vi "_Get FPGA Info.vi"(4 "error in":errorcluster) -> (0 "error out":errorcluster, 3 "Info":string)   [LabVIEW 2012]
uses:
  _RT Global.vi
  <vilib>/Utility/error.llb/Error Cluster From Error Code.vi
  <vilib>/rvi/errors/niLvFpgaAdjustHostInterfaceError.vi
  <vilib>/rvi/interface/nirviReadWriteControl/nirviReadWriteControl.xnode
  FPGA Bitfiles/FPGA9602.lvbitx
  NiFpgaLv.dll
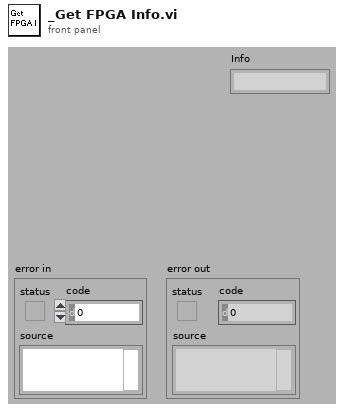
[diagram p1: front panel]
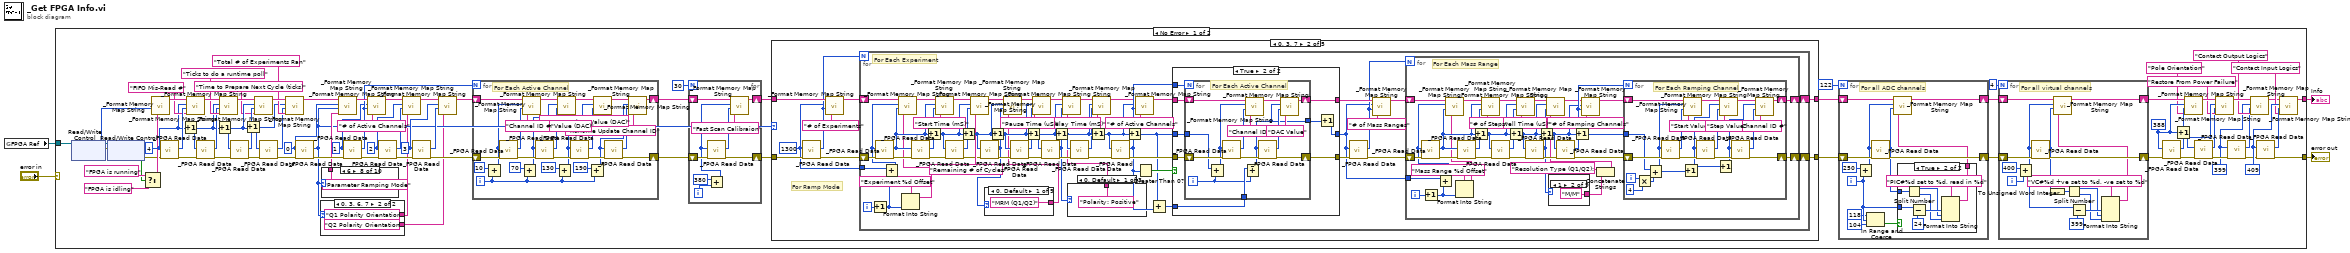
[diagram p0: block diagram]
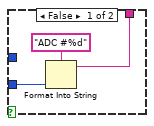
[diagram p2: hidden frame]
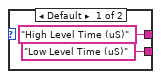
[diagram p3: hidden frame]
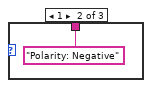
[diagram p5: hidden frame]
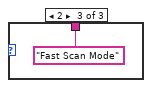
[diagram p6: hidden frame]
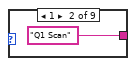
[diagram p7: hidden frame]
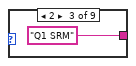
[diagram p8: hidden frame]
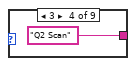
[diagram p9: hidden frame]
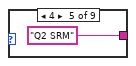
[diagram p10: hidden frame]
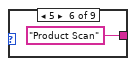
[diagram p11: hidden frame]
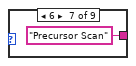
[diagram p12: hidden frame]
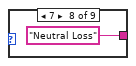
[diagram p13: hidden frame]
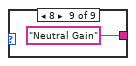
[diagram p14: hidden frame]
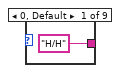
[diagram p15: hidden frame]
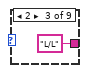
[diagram p16: hidden frame]
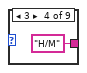
[diagram p17: hidden frame]
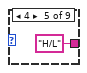
[diagram p18: hidden frame]
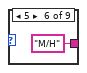
[diagram p19: hidden frame]
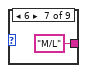
[diagram p20: hidden frame]
diagram:
  n1 = global read "_RT Global.vi" "FPGA Ref"() -> (w1:refnum<k20>)
  n2 = case shown="No Error" "error in" {
    selector: "error in" -> [_ w595]
    tunnel: [w6 w595] -> w3
    tunnel: w1 -> [w82 _]
    tunnel: [w5 _] -> w2
    frame No Error {
      w10 = u16 409 ("Address")
      w13 = u16 399 ("Address")
      w23 = u16 388 ("Address")
      w60 = u16 3 ("Address")
      w55 = u16 2 ("Address")
      w44 = u16 1 ("Address")
      w71 = u16 0 ("Address")
      w74 = u16 4 ("Address")
      n3 = xnode "Read/Write Control"("FPGA VI Reference In"=w82) -> ("FPGA VI Reference Out"=w84:refnum<k20>, "error out"=w83:errorcluster, "Version"=w80:u32)  [unwired: 1 in]
      n4 = xnode "Read/Write Control"("FPGA VI Reference In"=w84, "error in"=w83) -> ("error out"=w79:errorcluster, "Running"=w85:bool)  [unwired: 1 out]
      n5 = Select(t="FPGA is running", s=w85, f="FPGA is idling") -> (s? t:f=w81:string)
      n6 = call "_Format Memory Map String.vi"("User value"=w81, "Data"=w80) -> ("String Out"=w78:string)  [unwired: 2 in, 3 out]
      n7 = call "_FPGA Read Data.vi"("error in"=w79, "Address"=w74) -> ("error out"=w73:errorcluster, "Data"=w77:u32)  [unwired: 3 in, 1 out]
      n8 = Increment(x=w74) -> (x+1=w66:u16)
      n9 = call "_Format Memory Map String.vi"("User value"="FIFO Mis-Read #", "Data"=w77, "Address"=w74, "String In"=w78) -> ("String Out"=w75:string)  [unwired: 3 out]
      n10 = call "_FPGA Read Data.vi"("error in"=w73, "Address"=w66) -> ("error out"=w69:errorcluster, "Data"=w68:u32)  [unwired: 3 in, 1 out]
      n11 = Increment(x=w66) -> (x+1=w64:u16)
      n12 = call "_Format Memory Map String.vi"("User value"="Ticks to do a runtime poll", "Data"=w68, "Address"=w66, "String In"=w75) -> ("String Out"=w70:string)  [unwired: 3 out]
      n13 = call "_FPGA Read Data.vi"("error in"=w69, "Address"=w64) -> ("error out"=w65:errorcluster, "Data"=w67:u32)  [unwired: 3 in, 1 out]
      n14 = Increment(x=w64) -> (x+1=w45:u16)
      n15 = call "_Format Memory Map String.vi"("User value"="Time to Prepare Next Cycle (ticks)", "Data"=w67, "Address"=w64, "String In"=w70) -> ("String Out"=w62:string)  [unwired: 3 out]
      n16 = call "_FPGA Read Data.vi"("error in"=w65, "Address"=w45) -> ("error out"=w42:errorcluster, "Data"=w46:u32)  [unwired: 3 in, 1 out]
      n17 = call "_Format Memory Map String.vi"("User value"="Total # of Experiments Ran", "Data"=w46, "Address"=w45, "String In"=w62) -> ("String Out"=w41:string)  [unwired: 3 out]
      n18 = call "_FPGA Read Data.vi"("error in"=w42, "Address"=w71) -> ("error out"=w50:errorcluster, "Data"=w40:u32)  [unwired: 3 in, 1 out]
      n19 = case shown="0, 3, 6, 7" w40 {
        tunnel: ["High Level Time (uS)" ("User value") "Q1 Polarity Orientation" ("User value")] -> w39
        tunnel: ["Low Level Time (uS)" ("User value") "Q2 Polarity Orientation" ("User value")] -> w38
        frame Default {
        }
        frame 0, 3, 6, 7 {
        }
      }
      n20 = case shown="6" w40 {
        tunnel: ["Unknown Mode" ("User value") "Dual or Ramp Mode" ("User value") "Single Mode" ("User value") "Dual Mode" ("User value") "Ramp Mode" ("User value") "ADC Mode" ("User value") "Oscillator Mode" ("User value") "Parameter Ramping Mode" ("User value") "LC Sync Mode" ("User value") "Set PIC Mode" ("User value")] -> w43
        frame Default {
        }
        frame 0 {
        }
        frame 1 {
        }
        frame 2 {
        }
        frame 3 {
        }
        frame 4 {
        }
        frame 5 {
        }
        frame 6 {
        }
        frame 7 {
        }
        frame 8 {
        }
      }
      n21 = call "_Format Memory Map String.vi"("User value"=w43, "Data"=w40, "Address"=w71, "String In"=w41) -> ("String Out"=w51:string)  [unwired: 3 out]
      n22 = call "_FPGA Read Data.vi"("error in"=w50, "Address"=w44) -> ("error out"=w54:errorcluster, "Data"=w47:u32)  [unwired: 3 in, 1 out]
      n23 = call "_Format Memory Map String.vi"("User value"="# of Active Channels", "Data"=w47, "Address"=w44, "String In"=w51) -> ("String Out"=w56:string)  [unwired: 3 out]
      n24 = call "_FPGA Read Data.vi"("error in"=w54, "Address"=w55) -> ("error out"=w57:errorcluster, "Data"=w53:u32)  [unwired: 3 in, 1 out]
      n25 = call "_Format Memory Map String.vi"("User value"=w39, "Data"=w53, "Address"=w55, "String In"=w56) -> ("String Out"=w58:string)  [unwired: 3 out]
      n26 = call "_FPGA Read Data.vi"("error in"=w57, "Address"=w60) -> ("error out"=w48:errorcluster, "Data"=w59:u32)  [unwired: 3 in, 1 out]
      n27 = call "_Format Memory Map String.vi"("User value"=w38, "Data"=w59, "Address"=w60, "String In"=w58) -> ("String Out"=w49:string)  [unwired: 3 out]
      n28 = for {
        N: w47 -> [_]
        shift-right: [w142] -> w34
        shift-left: w49 -> [w153]
        shift-right: [w158] -> w32
        shift-left: w48 -> [w161]
        i -> [w140]
        # "For Each Active Channel"
        n29 = Add(x=10 ("y"), y=w140) -> (x+y=w147:i32)
        n30 = call "_FPGA Read Data.vi"("error in"=w161, "Address"=w147) -> ("error out"=w160:errorcluster, "Data"=w152:u32)  [unwired: 3 in, 1 out]
        n31 = Add(x=70 ("y"), y=w140) -> (x+y=w148:i32)
        n32 = call "_Format Memory Map String.vi"("User value"="Channel ID #", "Data"=w152, "Address"=w147, "String In"=w153) -> ("String Out"=w156:string)  [unwired: 3 out]
        n33 = call "_FPGA Read Data.vi"("error in"=w160, "Address"=w148) -> ("error out"=w159:errorcluster, "Data"=w151:u32)  [unwired: 3 in, 1 out]
        n34 = Add(x=130 ("y"), y=w140) -> (x+y=w149:i32)
        n35 = call "_Format Memory Map String.vi"("User value"="High Value (DAC)", "Data"=w151, "Address"=w148, "String In"=w156) -> ("String Out"=w157:string)  [unwired: 3 out]
        n36 = call "_FPGA Read Data.vi"("error in"=w159, "Address"=w149) -> ("error out"=w158:errorcluster, "Data"=w150:u32)  [unwired: 3 in, 1 out]
        n37 = Add(x=190 ("y"), y=w140) -> (x+y=w139:i32)
        n38 = call "_Format Memory Map String.vi"("User value"="Low / Runtime Value (DAC)", "Data"=w150, "Address"=w149, "String In"=w157) -> ("String Out"=w143:string)  [unwired: 3 out]
        n39 = call "_FPGA Read Data.vi"("Address"=w139) -> ("Data"=w146:u32)  [unwired: 4 in, 2 out]
        n40 = call "_Format Memory Map String.vi"("User value"="Runtime Update Channel ID", "Data"=w146, "Address"=w139, "String In"=w143) -> ("String Out"=w142:string)  [unwired: 3 out]
      }
      n41 = for {
        N: 30 -> [_]
        shift-right: [w111] -> w33
        shift-left: w34 -> [w110]
        shift-right: [w104] -> w31
        shift-left: w32 -> [w109]
        i -> [w107]
        n42 = Add(x=380 ("y"), y=w107) -> (x+y=w106:i32)
        n43 = call "_FPGA Read Data.vi"("error in"=w109, "Address"=w106) -> ("error out"=w104:errorcluster, "Data"=w105:u32)  [unwired: 3 in, 1 out]
        n44 = call "_Format Memory Map String.vi"("User value"="Fast Scan Calibraion", "Data"=w105, "Address"=w106, "String In"=w110) -> ("String Out"=w111:string)  [unwired: 3 out]
      }
      n45 = case shown="0, 3, 7" w40 {
        tunnel: w31 -> [w165 w175 w384 w500 w550]
        tunnel: w33 -> [w166 w174 w383 w499 w549]
        tunnel: [w165 w169 w380 w502 w552] -> w35
        tunnel: [w166 w168 w379 w503 w536] -> w36
        frame Default {
        }
        frame 0, 3, 7 {
          w167 = u16 1300 ("Address")
          # "For Ramp Mode"
          n46 = call "_FPGA Read Data.vi"("error in"=w175, "Address"=w167) -> ("error out"=w170:errorcluster, "Data"=w171:u32)  [unwired: 3 in, 1 out]
          n47 = call "_Format Memory Map String.vi"("User value"="# of Experiments", "Data"=w171, "Address"=w167, "String In"=w174) -> ("String Out"=w172:string)  [unwired: 3 out]
          n48 = for {
            N: w171 -> [_]
            shift-right: [w208] -> w168
            shift-left: w172 -> [w231]
            shift-right: [w207] -> w169
            shift-left: w170 -> [w232]
            tunnel: w167 -> [w203]
            i -> [w205]
            # "For Each Experiment"
            n49 = Increment(x=w205) -> (x+1=w204:i32)
            n50 = Add(x=w203, y=w204) -> (x+y=w230:i32)
            n51 = call "_FPGA Read Data.vi"("error in"=w232, "Address"=w230) -> ("error out"=w228:errorcluster, "Data"=w202:u32)  [unwired: 3 in, 1 out]
            n52 = Format Into String(format string="Experiment %d Offset" ("User value"), w204) -> (resulting string=w197:string)  [unwired: 2 in, 1 out]
            n53 = call "_Format Memory Map String.vi"("User value"=w197, "Data"=w202, "Address"=w230, "String In"=w231) -> ("String Out"=w227:string)  [unwired: 3 out]
            n54 = call "_FPGA Read Data.vi"("error in"=w228, "Address"=w202) -> ("error out"=w222:errorcluster, "Data"=w226:u32)  [unwired: 3 in, 1 out]
            n55 = Increment(x=w202) -> (x+1=w220:u32)
            n56 = call "_Format Memory Map String.vi"("User value"="Start Time (mS)", "Data"=w226, "Address"=w202, "String In"=w227) -> ("String Out"=w221:string)  [unwired: 3 out]
            n57 = call "_FPGA Read Data.vi"("error in"=w222, "Address"=w220) -> ("error out"=w192:errorcluster, "Data"=w223:u32)  [unwired: 3 in, 1 out]
            n58 = Increment(x=w220) -> (x+1=w191:u32)
            n59 = call "_Format Memory Map String.vi"("User value"="Remaining # of Cycles", "Data"=w223, "Address"=w220, "String In"=w221) -> ("String Out"=w195:string)  [unwired: 3 out]
            n60 = call "_FPGA Read Data.vi"("error in"=w192, "Address"=w191) -> ("error out"=w193:errorcluster, "Data"=w179:u32)  [unwired: 3 in, 1 out]
            n61 = case shown="0, Default" w179 {
              tunnel: ["MRM (Q1/Q2)" "Q1 Scan" "Q1 SRM" "Q2 Scan" "Q2 SRM" "Product Scan" "Precursor Scan" "Neutral Loss" "Neutral Gain"] -> w178
              frame 0, Default {
              }
              frame 1 {
              }
              frame 2 {
              }
              frame 3 {
              }
              frame 4 {
              }
              frame 5 {
              }
              frame 6 {
              }
              frame 7 {
              }
              frame 8 {
              }
            }
            n62 = Increment(x=w191) -> (x+1=w194:u32)
            n63 = call "_Format Memory Map String.vi"("User value"=w178, "Data"=w179, "Address"=w191, "String In"=w195) -> ("String Out"=w196:string)  [unwired: 3 out]
            n64 = call "_FPGA Read Data.vi"("error in"=w193, "Address"=w194) -> ("error out"=w186:errorcluster, "Data"=w199:u32)  [unwired: 3 in, 1 out]
            n65 = Increment(x=w194) -> (x+1=w183:u32)
            n66 = call "_Format Memory Map String.vi"("User value"="Pause Time (uS)", "Data"=w199, "Address"=w194, "String In"=w196) -> ("String Out"=w190:string)  [unwired: 3 out]
            n67 = call "_FPGA Read Data.vi"("error in"=w186, "Address"=w183) -> ("error out"=w185:errorcluster, "Data"=w177:u32)  [unwired: 3 in, 1 out]
            n68 = Increment(x=w183) -> (x+1=w182:u32)
            n69 = case shown="0, Default" w177 {
              tunnel: ["Polarity: Positive" ("User value") "Polarity: Negative" ("User value") "Fast Scan Mode" ("User value")] -> w176
              frame 0, Default {
              }
              frame 1 {
              }
              frame 2 {
              }
            }
            n70 = call "_Format Memory Map String.vi"("User value"=w176, "Data"=w177, "Address"=w183, "String In"=w190) -> ("String Out"=w189:string)  [unwired: 3 out]
            n71 = call "_FPGA Read Data.vi"("error in"=w185, "Address"=w182) -> ("error out"=w184:errorcluster, "Data"=w181:u32)  [unwired: 3 in, 1 out]
            n72 = Increment(x=w182) -> (x+1=w187:u32)
            n73 = call "_Format Memory Map String.vi"("User value"="Delay Time (mS)", "Data"=w181, "Address"=w182, "String In"=w189) -> ("String Out"=w188:string)  [unwired: 3 out]
            n74 = call "_FPGA Read Data.vi"("error in"=w184, "Address"=w187) -> ("error out"=w216:errorcluster, "Data"=w201:u32)  [unwired: 3 in, 1 out]
            n75 = Increment(x=w187) -> (x+1=w215:u32)
            n76 = call "_Format Memory Map String.vi"("User value"="# of Active Channels", "Data"=w201, "Address"=w187, "String In"=w188) -> ("String Out"=w217:string)  [unwired: 3 out]
            n77 = Greater Than 0?(x=w201) -> (x > 0?=w218:bool)
            n78 = Add(x=w215, y=w201) -> (x+y=w214:u32)
            n79 = case shown="True" w218 {
              tunnel: w215 -> [w311 w316]
              tunnel: w217 -> [w312 w321]
              tunnel: w216 -> [w310 w319]
              tunnel: w201 -> [_ w320]
              tunnel: [w312 w318] -> w212
              tunnel: [w311 w314] -> w200
              tunnel: [w310 w317] -> w213
              tunnel: w214 -> [_ w313]
              frame False {
              }
              frame True {
                n80 = for {
                  N: w320 -> [_]
                  shift-right: [w326] -> w318
                  shift-left: w321 -> [w331]
                  shift-right: [w325] -> w317
                  shift-left: w319 -> [w336]
                  tunnel: w316 -> [w327]
                  tunnel: [w324] -> w315
                  tunnel: w313 -> [w323]
                  i -> [w322]
                  # "For Each Active Channel"
                  n81 = Add(x=w327, y=w322) -> (x+y=w328:u32)
                  n82 = call "_FPGA Read Data.vi"("error in"=w336, "Address"=w328) -> ("error out"=w335:errorcluster, "Data"=w330:u32)  [unwired: 3 in, 1 out]
                  n83 = Add(x=w323, y=w322) -> (x+y=w324:u32)
                  n84 = call "_Format Memory Map String.vi"("User value"="Channel ID #", "Data"=w330, "Address"=w328, "String In"=w331) -> ("String Out"=w334:string)  [unwired: 3 out]
                  n85 = call "_FPGA Read Data.vi"("error in"=w335, "Address"=w324) -> ("error out"=w325:errorcluster, "Data"=w329:u32)  [unwired: 3 in, 1 out]
                  n86 = call "_Format Memory Map String.vi"("User value"="DAC Value", "Data"=w329, "Address"=w324, "String In"=w334) -> ("String Out"=w326:string)  [unwired: 3 out]
                }
                n87 = Increment(x=w315) -> (x+1=w314:u32)
              }
            }
            n88 = call "_FPGA Read Data.vi"("error in"=w213, "Address"=w200) -> ("error out"=w209:errorcluster, "Data"=w206:u32)  [unwired: 3 in, 1 out]
            n89 = call "_Format Memory Map String.vi"("User value"="# of Mass Ranges", "Data"=w206, "Address"=w200, "String In"=w212) -> ("String Out"=w210:string)  [unwired: 3 out]
            n90 = for {
              N: w206 -> [_]
              shift-right: [w260] -> w208
              shift-left: w210 -> [w277]
              shift-right: [w259] -> w207
              shift-left: w209 -> [w278]
              tunnel: w200 -> [w279]
              i -> [w258]
              # "For Each Mass Range"
              n91 = Increment(x=w258) -> (x+1=w257:i32)
              n92 = Add(x=w279, y=w257) -> (x+y=w256:u32)
              n93 = call "_FPGA Read Data.vi"("error in"=w278, "Address"=w256) -> ("error out"=w266:errorcluster, "Data"=w265:u32)  [unwired: 3 in, 1 out]
              n94 = Format Into String(format string="Mass Range %d Offset" ("User value"), w257) -> (resulting string=w255:string)  [unwired: 2 in, 1 out]
              n95 = call "_Format Memory Map String.vi"("User value"=w255, "Data"=w265, "Address"=w256, "String In"=w277) -> ("String Out"=w267:string)  [unwired: 3 out]
              n96 = call "_FPGA Read Data.vi"("error in"=w266, "Address"=w265) -> ("error out"=w271:errorcluster, "Data"=w275:u32)  [unwired: 3 in, 1 out]
              n97 = Increment(x=w265) -> (x+1=w269:u32)
              n98 = call "_Format Memory Map String.vi"("User value"="# of Steps", "Data"=w275, "Address"=w265, "String In"=w267) -> ("String Out"=w270:string)  [unwired: 3 out]
              n99 = call "_FPGA Read Data.vi"("error in"=w271, "Address"=w269) -> ("error out"=w251:errorcluster, "Data"=w272:u32)  [unwired: 3 in, 1 out]
              n100 = Increment(x=w269) -> (x+1=w250:u32)
              n101 = call "_Format Memory Map String.vi"("User value"="Dwell Time (uS)", "Data"=w272, "Address"=w269, "String In"=w270) -> ("String Out"=w254:string)  [unwired: 3 out]
              n102 = call "_FPGA Read Data.vi"("error in"=w251, "Address"=w250) -> ("error out"=w252:errorcluster, "Data"=w248:u32)  [unwired: 3 in, 1 out]
              n103 = Increment(x=w250) -> (x+1=w249:u32)
              n104 = case shown="1" w248 {
                tunnel: ["H/H" "M/M" "L/L" "H/M" "H/L" "M/H" "M/L" "L/H" "L/M"] -> w247
                frame 0, Default {
                }
                frame 1 {
                }
                frame 2 {
                }
                frame 3 {
                }
                frame 4 {
                }
                frame 5 {
                }
                frame 6 {
                }
                frame 7 {
                }
                frame 8 {
                }
              }
              n105 = call "_FPGA Read Data.vi"("error in"=w252, "Address"=w249) -> ("error out"=w263:errorcluster, "Data"=w262:u32)  [unwired: 3 in, 1 out]
              n106 = Increment(x=w249) -> (x+1=w261:u32)
              n107 = Concatenate Strings("Resolution Type (Q1/Q2): " ("User value"), w247) -> (w245:string)
              n108 = call "_Format Memory Map String.vi"("User value"=w245, "Data"=w248, "Address"=w250, "String In"=w254) -> ("String Out"=w253:string)  [unwired: 3 out]
              n109 = call "_Format Memory Map String.vi"("User value"="# of Ramping Channels", "Data"=w262, "Address"=w249, "String In"=w253) -> ("String Out"=w264:string)  [unwired: 3 out]
              n110 = for {
                N: w262 -> [_]
                shift-right: [w292] -> w260
                shift-left: w264 -> [w297]
                shift-right: [w303] -> w259
                shift-left: w263 -> [w306]
                tunnel: w261 -> [w291]
                i -> [w308]
                # "For Each Ramping Channel"
                n111 = Multiply(x=w308, y=4) -> (x*y=w307:i32)
                n112 = Add(x=w291, y=w307) -> (x+y=w290:u32)
                n113 = call "_FPGA Read Data.vi"("error in"=w306, "Address"=w290) -> ("error out"=w305:errorcluster, "Data"=w296:u32)  [unwired: 3 in, 1 out]
                n114 = Increment(x=w290) -> (x+1=w289:u32)
                n115 = call "_Format Memory Map String.vi"("User value"="Start Value", "Data"=w296, "Address"=w290, "String In"=w297) -> ("String Out"=w300:string)  [unwired: 3 out]
                n116 = call "_FPGA Read Data.vi"("error in"=w305, "Address"=w289) -> ("error out"=w304:errorcluster, "Data"=w295:u32)  [unwired: 3 in, 1 out]
                n117 = Increment(x=w289) -> (x+1=w293:u32)
                n118 = call "_Format Memory Map String.vi"("User value"="Step Value", "Data"=w295, "Address"=w289, "String In"=w300) -> ("String Out"=w302:string)  [unwired: 3 out]
                n119 = call "_FPGA Read Data.vi"("error in"=w304, "Address"=w293) -> ("error out"=w303:errorcluster, "Data"=w294:u32)  [unwired: 3 in, 1 out]
                n120 = call "_Format Memory Map String.vi"("User value"="Channel ID #", "Data"=w294, "Address"=w293, "String In"=w302) -> ("String Out"=w292:string)  [unwired: 3 out]
              }
            }
          }
        }
        frame 6 {
          w359 = u16 1300 ("Address")
          # "For Ramping Parameter Mode"
          n121 = call "_FPGA Read Data.vi"("error in"=w384, "Address"=w359) -> ("error out"=w361:errorcluster, "Data"=w381:u32)  [unwired: 3 in, 1 out]
          n122 = Increment(x=w359) -> (x+1=w376:u16)
          n123 = call "_Format Memory Map String.vi"("User value"="# of Experiments", "Data"=w381, "Address"=w359, "String In"=w383) -> ("String Out"=w360:string)  [unwired: 3 out]
          n124 = call "_FPGA Read Data.vi"("error in"=w361, "Address"=w376) -> ("error out"=w363:errorcluster, "Data"=w377:u32)  [unwired: 3 in, 1 out]
          n125 = Increment(x=w376) -> (x+1=w362:u16)
          n126 = call "_Format Memory Map String.vi"("User value"="Remaining # of Cycles", "Data"=w377, "Address"=w376, "String In"=w360) -> ("String Out"=w366:string)  [unwired: 3 out]
          n127 = call "_FPGA Read Data.vi"("error in"=w363, "Address"=w362) -> ("error out"=w364:errorcluster, "Data"=w349:u32)  [unwired: 3 in, 1 out]
          n128 = case shown="0, Default" w349 {
            tunnel: ["MRM (Q1/Q2)" "Q1 Scan" "Q1 SRM" "Q2 Scan" "Q2 SRM" "Product Scan" "Precursor Scan" "Neutral Loss" "Neutral Gain"] -> w348
            frame 0, Default {
            }
            frame 1 {
            }
            frame 2 {
            }
            frame 3 {
            }
            frame 4 {
            }
            frame 5 {
            }
            frame 6 {
            }
            frame 7 {
            }
            frame 8 {
            }
          }
          n129 = Increment(x=w362) -> (x+1=w365:u16)
          n130 = call "_Format Memory Map String.vi"("User value"=w348, "Data"=w349, "Address"=w362, "String In"=w366) -> ("String Out"=w367:string)  [unwired: 3 out]
          n131 = call "_FPGA Read Data.vi"("error in"=w364, "Address"=w365) -> ("error out"=w352:errorcluster, "Data"=w369:u32)  [unwired: 3 in, 1 out]
          n132 = Increment(x=w365) -> (x+1=w351:u16)
          n133 = call "_Format Memory Map String.vi"("User value"="Pause Time (uS)", "Data"=w369, "Address"=w365, "String In"=w367) -> ("String Out"=w354:string)  [unwired: 3 out]
          n134 = call "_FPGA Read Data.vi"("error in"=w352, "Address"=w351) -> ("error out"=w350:errorcluster, "Data"=w346:u32)  [unwired: 3 in, 1 out]
          n135 = case shown="2" w346 {
            tunnel: ["Polarity: Positive" ("User value") "Polarity: Negative" ("User value") "Fast Scan Mode" ("User value")] -> w345
            frame 0, Default {
            }
            frame 1 {
            }
            frame 2 {
            }
          }
          n136 = call "_Format Memory Map String.vi"("User value"=w345, "Data"=w346, "Address"=w351, "String In"=w354) -> ("String Out"=w353:string)  [unwired: 3 out]
          n137 = Increment(x=w351) -> (x+1=w347:u16)
          n138 = call "_FPGA Read Data.vi"("error in"=w350, "Address"=w347) -> ("error out"=w357:errorcluster, "Data"=w370:u32)  [unwired: 3 in, 1 out]
          n139 = Increment(x=w347) -> (x+1=w356:u16)
          n140 = call "_Format Memory Map String.vi"("User value"="Delay Time (mS)", "Data"=w370, "Address"=w347, "String In"=w353) -> ("String Out"=w358:string)  [unwired: 3 out]
          n141 = call "_FPGA Read Data.vi"("error in"=w357, "Address"=w356) -> ("error out"=w342:errorcluster, "Data"=w338:u32)  [unwired: 3 in, 1 out]
          n142 = Increment(x=w356) -> (x+1=w341:u16)
          n143 = call "_Format Memory Map String.vi"("User value"="Number of Active Channels", "Data"=w338, "Address"=w356, "String In"=w358) -> ("String Out"=w344:string)  [unwired: 3 out]
          n144 = Greater Than 0?(x=w338) -> (x > 0?=w337:bool)
          n145 = case shown="True" w337 {
            tunnel: w338 -> [_ w394]
            tunnel: w344 -> [w385 w393]
            tunnel: [w385 w392] -> w343
            tunnel: w342 -> [w386 w391]
            tunnel: w341 -> [w387 w390]
            tunnel: [w387 w389] -> w340
            tunnel: [w386 w388] -> w339
            frame False {
            }
            frame True {
              n146 = for {
                N: w394 -> [_]
                shift-right: [w401] -> w392
                shift-left: w393 -> [w405]
                shift-right: [w411] -> w388
                shift-left: w391 -> [w414]
                tunnel: w390 -> [w400]
                tunnel: [w395] -> w389
                i -> [w416]
                # "For Each Ramping Channel"
                n147 = Multiply(x=w416, y=4) -> (x*y=w415:i32)
                n148 = Add(x=w400, y=w415) -> (x+y=w399:i32)
                n149 = call "_FPGA Read Data.vi"("error in"=w414, "Address"=w399) -> ("error out"=w413:errorcluster, "Data"=w404:u32)  [unwired: 3 in, 1 out]
                n150 = Increment(x=w399) -> (x+1=w398:i32)
                n151 = call "_Format Memory Map String.vi"("User value"="Start Value", "Data"=w404, "Address"=w399, "String In"=w405) -> ("String Out"=w408:string)  [unwired: 3 out]
                n152 = call "_FPGA Read Data.vi"("error in"=w413, "Address"=w398) -> ("error out"=w412:errorcluster, "Data"=w403:u32)  [unwired: 3 in, 1 out]
                n153 = Increment(x=w398) -> (x+1=w397:i32)
                n154 = call "_Format Memory Map String.vi"("User value"="Step Value", "Data"=w403, "Address"=w398, "String In"=w408) -> ("String Out"=w410:string)  [unwired: 3 out]
                n155 = call "_FPGA Read Data.vi"("error in"=w412, "Address"=w397) -> ("error out"=w411:errorcluster, "Data"=w402:u32)  [unwired: 3 in, 1 out]
                n156 = Add(x=w397, y=2) -> (x+y=w395:i32)
                n157 = call "_Format Memory Map String.vi"("User value"="Channel ID #", "Data"=w402, "Address"=w397, "String In"=w410) -> ("String Out"=w401:string)  [unwired: 3 out]
              }
            }
          }
          n158 = call "_FPGA Read Data.vi"("error in"=w339, "Address"=w340) -> ("error out"=w372:errorcluster, "Data"=w371:u32)  [unwired: 3 in, 1 out]
          n159 = call "_Format Memory Map String.vi"("User value"="# of Mass Ranges", "Data"=w371, "Address"=w340, "String In"=w343) -> ("String Out"=w373:string)  [unwired: 3 out]
          n160 = for {
            N: w371 -> [_]
            shift-right: [w445] -> w379
            shift-left: w373 -> [w462]
            shift-right: [w444] -> w380
            shift-left: w372 -> [w463]
            tunnel: w340 -> [w464]
            i -> [w443]
            # "For Each Mass Range"
            n161 = Increment(x=w443) -> (x+1=w442:i32)
            n162 = Add(x=w464, y=w442) -> (x+y=w441:i32)
            n163 = call "_FPGA Read Data.vi"("error in"=w463, "Address"=w441) -> ("error out"=w451:errorcluster, "Data"=w450:u32)  [unwired: 3 in, 1 out]
            n164 = Format Into String(format string="Mass Range %d Offset" ("User value"), w442) -> (resulting string=w440:string)  [unwired: 2 in, 1 out]
            n165 = call "_Format Memory Map String.vi"("User value"=w440, "Data"=w450, "Address"=w441, "String In"=w462) -> ("String Out"=w452:string)  [unwired: 3 out]
            n166 = call "_FPGA Read Data.vi"("error in"=w451, "Address"=w450) -> ("error out"=w456:errorcluster, "Data"=w460:u32)  [unwired: 3 in, 1 out]
            n167 = Increment(x=w450) -> (x+1=w454:u32)
            n168 = call "_Format Memory Map String.vi"("User value"="# of Steps", "Data"=w460, "Address"=w450, "String In"=w452) -> ("String Out"=w455:string)  [unwired: 3 out]
            n169 = call "_FPGA Read Data.vi"("error in"=w456, "Address"=w454) -> ("error out"=w436:errorcluster, "Data"=w457:u32)  [unwired: 3 in, 1 out]
            n170 = Increment(x=w454) -> (x+1=w435:u32)
            n171 = call "_Format Memory Map String.vi"("User value"="Dwell Time (uS)", "Data"=w457, "Address"=w454, "String In"=w455) -> ("String Out"=w439:string)  [unwired: 3 out]
            n172 = call "_FPGA Read Data.vi"("error in"=w436, "Address"=w435) -> ("error out"=w437:errorcluster, "Data"=w431:u32)  [unwired: 3 in, 1 out]
            n173 = Increment(x=w435) -> (x+1=w434:u32)
            n174 = case shown="0, Default" w431 {
              tunnel: ["H/H" "M/M" "L/L" "H/M" "H/L" "M/H" "M/L" "L/H" "L/M"] -> w433
              frame 0, Default {
              }
              frame 1 {
              }
              frame 2 {
              }
              frame 3 {
              }
              frame 4 {
              }
              frame 5 {
              }
              frame 6 {
              }
              frame 7 {
              }
              frame 8 {
              }
            }
            n175 = call "_FPGA Read Data.vi"("error in"=w437, "Address"=w434) -> ("error out"=w448:errorcluster, "Data"=w447:u32)  [unwired: 3 in, 1 out]
            n176 = Increment(x=w434) -> (x+1=w446:u32)
            n177 = Concatenate Strings("Resolution Type (Q1/Q2): " ("User value"), w433) -> (w430:string)
            n178 = call "_Format Memory Map String.vi"("User value"=w430, "Data"=w431, "Address"=w435, "String In"=w439) -> ("String Out"=w438:string)  [unwired: 3 out]
            n179 = call "_Format Memory Map String.vi"("User value"="# of Ramping Channels", "Data"=w447, "Address"=w434, "String In"=w438) -> ("String Out"=w449:string)  [unwired: 3 out]
            n180 = for {
              N: w447 -> [_]
              shift-right: [w477] -> w445
              shift-left: w449 -> [w482]
              shift-right: [w488] -> w444
              shift-left: w448 -> [w491]
              tunnel: w446 -> [w476]
              i -> [w493]
              # "For Each Ramping Channel"
              n181 = Multiply(x=w493, y=4) -> (x*y=w492:i32)
              n182 = Add(x=w476, y=w492) -> (x+y=w475:u32)
              n183 = call "_FPGA Read Data.vi"("error in"=w491, "Address"=w475) -> ("error out"=w490:errorcluster, "Data"=w481:u32)  [unwired: 3 in, 1 out]
              n184 = Increment(x=w475) -> (x+1=w474:u32)
              n185 = call "_Format Memory Map String.vi"("User value"="Start Value", "Data"=w481, "Address"=w475, "String In"=w482) -> ("String Out"=w485:string)  [unwired: 3 out]
              n186 = call "_FPGA Read Data.vi"("error in"=w490, "Address"=w474) -> ("error out"=w489:errorcluster, "Data"=w480:u32)  [unwired: 3 in, 1 out]
              n187 = Increment(x=w474) -> (x+1=w478:u32)
              n188 = call "_Format Memory Map String.vi"("User value"="Step Value", "Data"=w480, "Address"=w474, "String In"=w485) -> ("String Out"=w487:string)  [unwired: 3 out]
              n189 = call "_FPGA Read Data.vi"("error in"=w489, "Address"=w478) -> ("error out"=w488:errorcluster, "Data"=w479:u32)  [unwired: 3 in, 1 out]
              n190 = call "_Format Memory Map String.vi"("User value"="Channel ID #", "Data"=w479, "Address"=w478, "String In"=w487) -> ("String Out"=w477:string)  [unwired: 3 out]
            }
          }
        }
        frame 5 {
          w497 = u16 7 ("Address")
          w507 = 8 ("y")
          # "For Oscillator Mode"
          n191 = call "_FPGA Read Data.vi"("error in"=w500, "Address"=w497) -> ("error out"=w501:errorcluster, "Data"=w496:u32)  [unwired: 3 in, 1 out]
          n192 = case shown="0, Default" w496 {
            tunnel: ["Programming for Q1-FREQ" ("User value") "Programming for Q3-FREQ" ("User value") "Programming for MP1-FREQ" ("User value")] -> w495
            frame 0, Default {
            }
            frame 1 {
            }
            frame 2 {
            }
          }
          n193 = call "_Format Memory Map String.vi"("User value"=w495, "Data"=w496, "Address"=w497, "String In"=w499) -> ("String Out"=w498:string)  [unwired: 3 out]
          n194 = call "_FPGA Read Data.vi"("error in"=w501, "Address"=w507) -> ("error out"=w525:errorcluster, "Data"=w512:u32)  [unwired: 3 in, 1 out]
          n195 = Increment(x=w507) -> (x+1=w505:i32)
          n196 = call "_FPGA Read Data.vi"("error in"=w525, "Address"=w505) -> ("error out"=w502:errorcluster, "Data"=w504:u32)  [unwired: 3 in, 1 out]
          n197 = Split Number(x=w512) -> (hi(x)=w522:u16, lo(x)=w521:u16)
          n198 = Split Number(x=w504) -> (hi(x)=w524:u16, lo(x)=w523:u16)
          n199 = Split Number(x=w524) -> (hi(x)=w518:u8, lo(x)=w517:u8)
          n200 = Split Number(x=w523) -> (hi(x)=w516:u8, lo(x)=w515:u8)
          n201 = Split Number(x=w522) -> (hi(x)=w520:u8, lo(x)=w519:u8)
          n202 = Split Number(x=w521) -> (hi(x)=w514:u8, lo(x)=w513:u8)
          n203 = Build Array(w520, w519, w518, w517, w516, w515, w514, w513) -> (w506:u8[])
          n204 = for {
            shift-right: [w535] -> w509
            shift-left: w498 -> [w534]
            tunnel: "Oscillator Register %d: %2.0xhex" ("User value") -> [w532]
            tunnel: w506 -> [w530] mode=indexing
            tunnel: w507 -> [w529]
            i -> [w533]
            n205 = Format Into String(format string=w532, w533, w530) -> (resulting string=w531:string)  [unwired: 2 in, 1 out]
            n206 = call "_Format Memory Map String.vi"("User value"=w531, "Data"=w530, "Address"=w529, "String In"=w534) -> ("String Out"=w535:string)  [unwired: 3 out]
          }
          n207 = Format Into String(format string="Oscillator frequency tuning word: %8.0xhex" ("User value"), w504) -> (resulting string=w508:string)  [unwired: 2 in, 1 out]
          n208 = call "_Format Memory Map String.vi"("User value"=w508, "Data"=w504, "Address"=w505, "String In"=w509) -> ("String Out"=w503:string)  [unwired: 3 out]
        }
        frame 8 {
          w547 = u16 7 ("Address")
          w555 = 8 ("y")
          # "For Set PIC Mode"
          n209 = call "_FPGA Read Data.vi"("error in"=w550, "Address"=w547) -> ("error out"=w551:errorcluster, "Data"=w546:u32)  [unwired: 3 in, 1 out]
          n210 = case shown="2" w546 {
            tunnel: ["Programming for PIC1" ("User value") "Programming for PIC2" ("User value") "Programming for PIC3" ("User value") "Programming for PIC4" ("User value")] -> w545
            frame 0, Default {
            }
            frame 1 {
            }
            frame 2 {
            }
            frame 3 {
            }
          }
          n211 = call "_Format Memory Map String.vi"("User value"=w545, "Data"=w546, "Address"=w547, "String In"=w549) -> ("String Out"=w548:string)  [unwired: 3 out]
          n212 = call "_FPGA Read Data.vi"("error in"=w551, "Address"=w555) -> ("error out"=w566:errorcluster, "Data"=w557:u32)  [unwired: 3 in, 1 out]
          n213 = Increment(x=w555) -> (x+1=w542:i32)
          n214 = call "_FPGA Read Data.vi"("error in"=w566, "Address"=w542) -> ("error out"=w552:errorcluster, "Data"=w553:u32)  [unwired: 3 in, 1 out]
          n215 = Split Number(x=w557) -> (hi(x)=w563:u16, lo(x)=w562:u16)
          n216 = Split Number(x=w553) -> (hi(x)=w565:u16, lo(x)=w564:u16)
          n217 = Split Number(x=w565) -> (hi(x)=w541:u8, lo(x)=w540:u8)
          n218 = Split Number(x=w564) -> (hi(x)=w539:u8, lo(x)=w538:u8)
          n219 = Split Number(x=w563) -> (hi(x)=w561:u8, lo(x)=w560:u8)
          n220 = Split Number(x=w562) -> (hi(x)=w559:u8, lo(x)=w558:u8)
          n221 = Build Array(w541, w540, w539, w538) -> (w537:u8[])
          n222 = Build Array(w561, w560, w559, w558) -> (w554:u8[])
          n223 = for {
            shift-right: [w584] -> w544
            shift-left: w548 -> [w583]
            tunnel: "PIC Instruction %d: %2.0xhex" ("User value") -> [w581]
            tunnel: w554 -> [w579] mode=indexing
            tunnel: w555 -> [w578]
            i -> [w582]
            n224 = Format Into String(format string=w581, w582, w579) -> (resulting string=w580:string)  [unwired: 2 in, 1 out]
            n225 = call "_Format Memory Map String.vi"("User value"=w580, "Data"=w579, "Address"=w578, "String In"=w583) -> ("String Out"=w584:string)  [unwired: 3 out]
          }
          n226 = for {
            shift-right: [w573] -> w536
            shift-left: w544 -> [w572]
            tunnel: "PIC Returns %d: %2.0xhex" ("User value") -> [w570]
            tunnel: w537 -> [w568] mode=indexing
            tunnel: w542 -> [w567]
            i -> [w571]
            n227 = Format Into String(format string=w570, w571, w568) -> (resulting string=w569:string)  [unwired: 2 in, 1 out]
            n228 = call "_Format Memory Map String.vi"("User value"=w569, "Data"=w568, "Address"=w567, "String In"=w572) -> ("String Out"=w573:string)  [unwired: 3 out]
          }
        }
      }
      n229 = for {
        N: 122 -> [_]
        shift-right: [w119] -> w28
        shift-left: w36 -> [w121]
        shift-right: [w118] -> w29
        shift-left: w35 -> [w122]
        i -> [w116]
        # "For all ADC channels"
        n230 = Add(x=250 ("y"), y=w116) -> (x+y=w120:i32)
        n231 = In Range and Coerce(upper limit=118, x=w116, lower limit=104) -> (In Range?=w113:bool)  [unwired: 1 out]
        n232 = call "_FPGA Read Data.vi"("error in"=w122, "Address"=w120) -> ("error out"=w118:errorcluster, "Data"=w112:u32)  [unwired: 3 in, 1 out]
        n233 = case shown="True" w113 {
          tunnel: [w125 w127] -> w117
          tunnel: w116 -> [w124 w134]
          tunnel: w112 -> [_ w132]
          frame False {
            n234 = Format Into String(format string="ADC #%d" ("User value"), w124) -> (resulting string=w125:string)  [unwired: 2 in, 1 out]
          }
          frame True {
            n235 = Split Number(x=w132) -> (hi(x)=w130:u16, lo(x)=w129:u16)
            n236 = Subtract(x=w134, y=24) -> (x-y=w131:i32)
            n237 = Format Into String(format string="PIC#%d set to %d, read in %d", w131, w130, w129) -> (resulting string=w127:string)  [unwired: 2 in, 1 out]
          }
        }
        n238 = call "_Format Memory Map String.vi"("User value"=w117, "Data"=w112, "Address"=w120, "String In"=w121) -> ("String Out"=w119:string)  [unwired: 3 out]
      }
      n239 = for {
        N: 4 -> [_]
        shift-right: [w99] -> w25
        shift-left: w28 -> [w100]
        shift-right: [w98] -> w26
        shift-left: w29 -> [w101]
        i -> [w96]
        # "For all virtual channels"
        n240 = Add(x=400 ("y"), y=w96) -> (x+y=w88:i32)
        n241 = call "_FPGA Read Data.vi"("error in"=w101, "Address"=w88) -> ("error out"=w98:errorcluster, "Data"=w95:u32)  [unwired: 3 in, 1 out]
        n242 = To Unsigned Word Integer(number=w95) -> (unsigned 16bit integer=w89:u16)
        n243 = Split Number(x=w89) -> (hi(x)=w92:u8, lo(x)=w91:u8)
        n244 = Subtract(x=w88, y=399) -> (x-y=w93:i32)
        n245 = Format Into String(format string="VC#%d +ve set to %d, -ve set to %d", w93, w92, w91) -> (resulting string=w97:string)  [unwired: 2 in, 1 out]
        n246 = call "_Format Memory Map String.vi"("User value"=w97, "Data"=w95, "Address"=w88, "String In"=w100) -> ("String Out"=w99:string)  [unwired: 3 out]
      }
      n247 = call "_FPGA Read Data.vi"("error in"=w26, "Address"=w23) -> ("error out"=w24:errorcluster, "Data"=w22:u32)  [unwired: 3 in, 1 out]
      n248 = Increment(x=w23) -> (x+1=w19:u16)
      n249 = call "_Format Memory Map String.vi"("User value"="Pole Orientation", "Data"=w22, "Address"=w23, "String In"=w25) -> ("String Out"=w20:string)  [unwired: 3 out]
      n250 = call "_FPGA Read Data.vi"("error in"=w24, "Address"=w19) -> ("error out"=w17:errorcluster, "Data"=w16:u32)  [unwired: 3 in, 1 out]
      n251 = call "_Format Memory Map String.vi"("User value"="Restore From Power Failure", "Data"=w16, "Address"=w19, "String In"=w20) -> ("String Out"=w15:string)  [unwired: 3 out]
      n252 = call "_FPGA Read Data.vi"("error in"=w17, "Address"=w13) -> ("error out"=w7:errorcluster, "Data"=w12:u32)  [unwired: 3 in, 1 out]
      n253 = call "_Format Memory Map String.vi"("User value"="Contact Output Logics", "Data"=w12, "Address"=w13, "String In"=w15) -> ("String Out"=w8:string)  [unwired: 3 out]
      n254 = call "_FPGA Read Data.vi"("error in"=w7, "Address"=w10) -> ("error out"=w6:errorcluster, "Data"=w11:u32)  [unwired: 3 in, 1 out]
      n255 = call "_Format Memory Map String.vi"("User value"="Contact Input Logics", "Data"=w11, "Address"=w10, "String In"=w8) -> ("String Out"=w5:string)  [unwired: 3 out]
    }
    frame Error {
    }
  }
  "error out" <- w3
  "Info" <- w2
